vi "Sort Media Types.vi"(11 "Parsed Types":T1[](array[typedef])) -> (3 "Sorted types":T1[](array[typedef]))   [LabVIEW 2011]
doc: "Sorts an array of media types according to the standard HTTP specification."
uses:
  Media Parameter.ctl
  Media Type.ctl
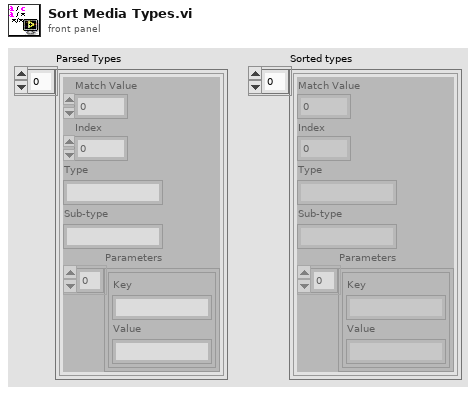
[diagram p1: front panel]
types:
  T1 = typedef "Media Type.ctl" = cluster{"Match Value":dbl, "Index":i32, "Type":string, "Sub-type":string, "Parameters":T2[]}
  T2 = typedef "Media Parameter.ctl" = cluster{"Key":string, "Value":string}
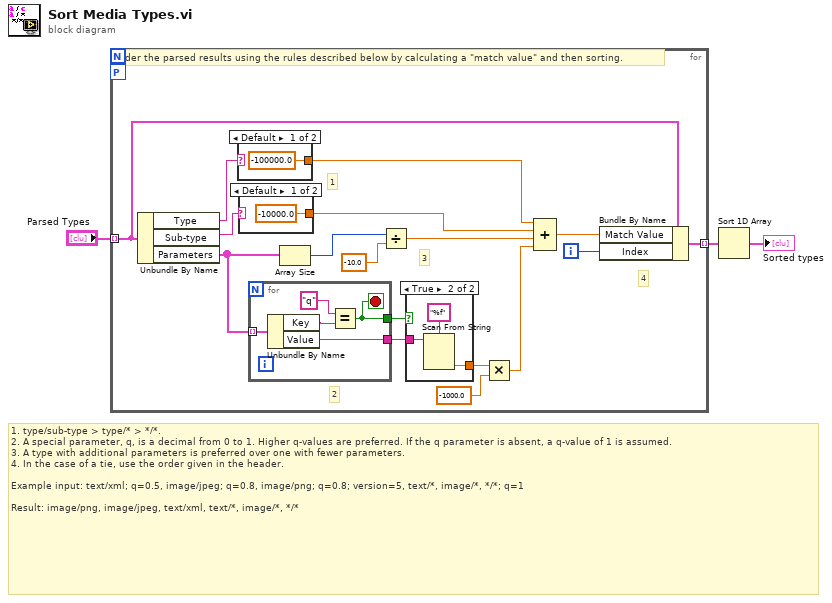
[diagram p0: block diagram]
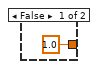
[diagram p2: hidden frame]
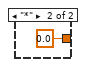
[diagram p3: hidden frame]
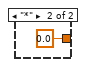
[diagram p4: hidden frame]
diagram:
  # "1. type/sub-type > type/* > */*.\n2. A special parameter, q, is a decimal from 0 to 1. Higher q-values are preferred. If the q parameter is absent, a q-value of 1 is assumed.\n3. A type with additional parameters is preferred over one with fewer parameters.\n4. In the case of a tie, use the order given in the header.\n\nExample input: text/xml; q=0.5, image/jpeg; q=0.8, image/png; q=0.8; version=5, text/*, image/*, */*; q=1\n\nResult: image/png, image/jpeg, text/xml, text/*, image/*, */*"
  n1 = for {
    tunnel: "Parsed Types" -> [w15] mode=indexing
    tunnel: [w8] -> w1 mode=indexing
    workers-P: _ -> [_]
    i -> [w9]
    # "4"
    # "3"
    # "2"
    # "1"
    # "Order the parsed results using the rules described below by calculating a \"match value\" and then sorting."
    n2 = Unbundle By Name(w15) -> ("Type"=w20:string, "Sub-type"=w19:string, "Parameters"=w18:T2[])
    n3 = case shown="Default" w20 {
      tunnel: [-100000.0 0.0] -> w11
      frame Default {
      }
      frame "*" {
      }
    }
    n4 = case shown="Default" w19 {
      tunnel: [-10000.0 0.0] -> w10
      frame Default {
      }
      frame "*" {
      }
    }
    n5 = for {
      tunnel: w18 -> [w29] mode=indexing
      tunnel: [w26] -> w17
      tunnel: [w25] -> w16
      stop <- w25 stop-if-true
      n6 = Unbundle By Name(w29) -> ("Key"=w28:string, "Value"=w26:string)
      n7 = Equal?(x="q", y=w28) -> (x = y?=w25:bool)
    }
    n8 = Array Size(array=w18) -> (size(s)=w12:i32)
    n9 = Divide(x=w12, y=-10.0 ("x")) -> (x/y=w7:dbl)
    n10 = case shown="True" w16 {
      tunnel: w17 -> [_ w24]
      tunnel: [1.0 w22] -> w14
      frame False {
      }
      frame True {
        n11 = Scan From String(format string="%f", input string=w24) -> (output 1=w22:dbl)  [unwired: 3 in, 3 out]
      }
    }
    n12 = Multiply(x=w14, y=-1000.0) -> (x*y=w5:dbl)
    n13 = Compound Arithmetic op=ADD(w11, w10, w7, w5) -> (w4:dbl)
    n14 = Bundle By Name(cluster=w15, "Match Value"=w4, "Index"=w9) -> (w8:T1)
  }
  n15 = Sort 1D Array(array=w1) -> (sorted array=→"Sorted types":T1[])
